vi "rearrangeElements.vi"(8 "error in (no error)":errorcluster, 11 "Topic in":refnum<class "Topic.lvclass">) -> (0 "error out":errorcluster, 3 "Topic out":refnum<class "Topic.lvclass">)   [LabVIEW 2013, in "Topic.lvclass"]
uses:
  Topic.lvclass
  Topic.lvclass/Topic.ctl
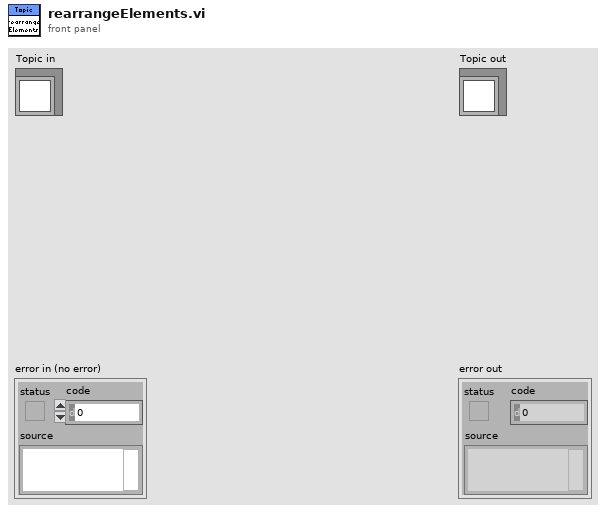
[diagram p1: front panel]
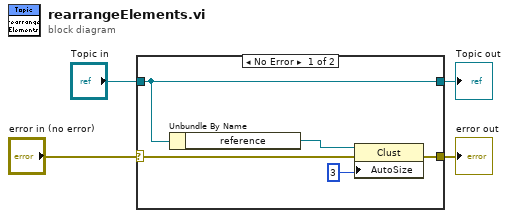
[diagram p0: block diagram]
diagram:
  n1 = case shown="No Error" "error in (no error)" {
    selector: "error in (no error)" -> [w6 w11]
    tunnel: [w5 w11] -> w3
    tunnel: [w8 w10] -> w1
    tunnel: "Topic in" -> [w8 w10]
    frame No Error {
      n2 = Unbundle By Name(w8) -> ("reference"=w7:refnum<vi>)
      n3 = property class="Clust"(reference=w7, error in=w6, "AutoSize"=u32 3 ("Auto Sizing")) -> (error out=w5:errorcluster)  [unwired: 1 out]
    }
    frame Error {
    }
  }
  "error out" <- w3
  "Topic out" <- w1
